vi "Main2.vi"() -> ()   [LabVIEW 2016]
panel:
  out "To send":i32
  out "Status":u16
  out "Pot 1":u16
  out "Pot 2":u16
  out "SW1 H":bool
  out "SW1 L":bool
  out "SW2 H":bool
  out "SW2 L":bool
  out "SW3 H":bool
  out "SW3 L":bool
  out "SW4 H":bool
  out "SW4 L":bool
  out "Read Status":bool[](array[boolean])
  in  "stop":bool
  out "FIFO notEmpty":bool
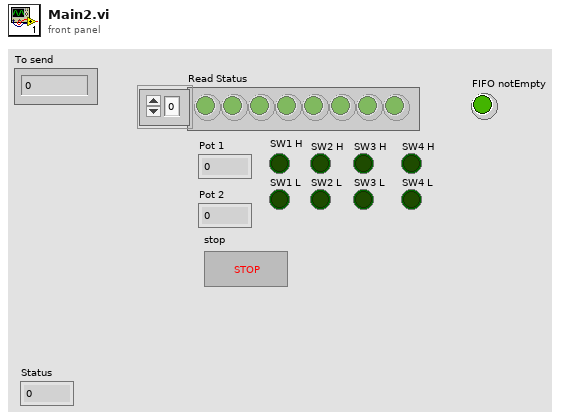
[diagram p1: front panel]
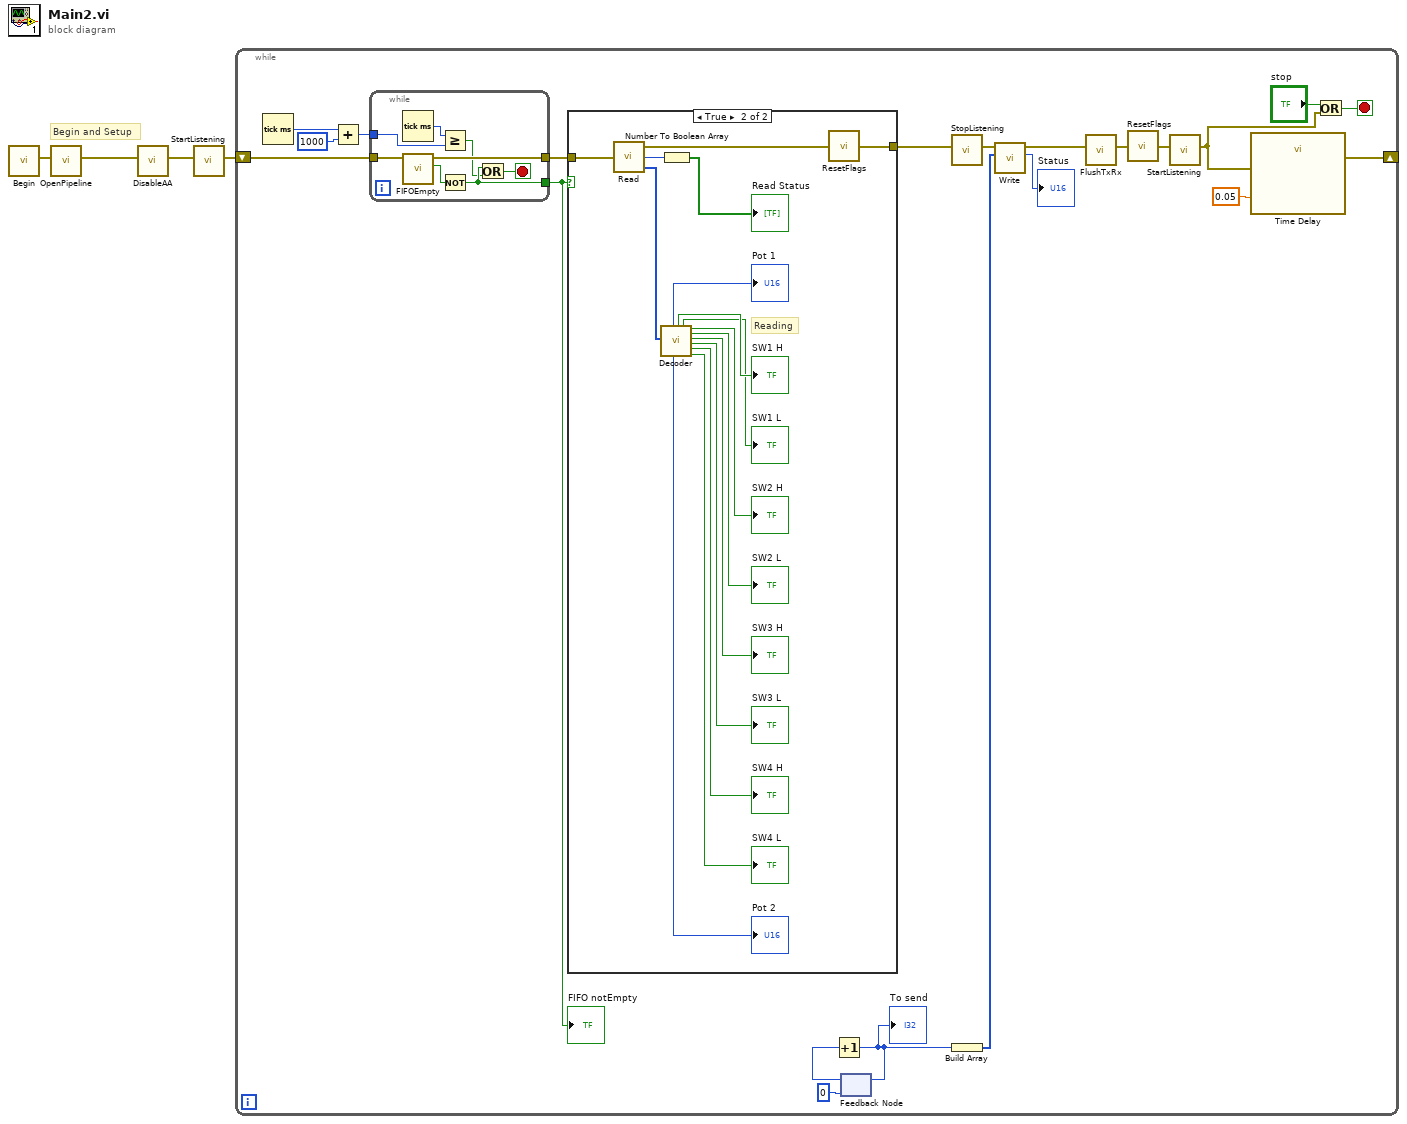
[diagram p0: block diagram]
diagram:
  # "Begin and Setup"
  n1 = call "Begin.vi"() -> ("error out"=w4:errorcluster)  [unwired: 11 in]
  n2 = call "OpenPipeline.vi"("error in (no error)"=w4) -> ("error out"=w3:errorcluster)  [unwired: 10 in]
  n3 = call "DisableAA.vi"("error in (no error)"=w3) -> ("error out"=w2:errorcluster)  [unwired: 10 in]
  n4 = call "StartListening.vi"("error in (no error)"=w2) -> ("error out"=w1:errorcluster)  [unwired: 10 in]
  n5 = while {
    shift-right: [w5] -> _
    shift-left: w1 -> [w22]
    stop <- w24 stop-if-true
    n6 = Tick Count (ms)() -> (millisecond timer value=w21:u32)
    n7 = Add(x=w21, y=u32 1000) -> (x+y=w19:u32)
    n8 = while {
      tunnel: [w33] -> w25
      tunnel: w22 -> [w32]
      tunnel: [w29] -> w8
      tunnel: w19 -> [w26]
      stop <- w30 stop-if-true
      n9 = Tick Count (ms)() -> (millisecond timer value=w28:u32)
      n10 = call "FIFOEmpty.vi"("error in (no error)"=w32) -> ("RX_EMPTY"=w31:bool, "error out"=w33:errorcluster)  [unwired: 9 in]
      n11 = Greater Or Equal?(x=w28, y=w26) -> (x >= y?=w27:bool)
      n12 = Not(x=w31) -> (.not. x?=w29:bool)
      n13 = Or(x=w29, y=w27) -> (x .or. y?=w30:bool)
    }
    "FIFO notEmpty" <- w8
    n14 = case shown="True" w8 {
      tunnel: w25 -> [w34 w36]
      tunnel: [w34 w35] -> w13
      frame False {
        # "Writing"
      }
      frame True {
        # "Reading"
        n15 = call "Read.vi"("error in (no error)"=w36) -> ("error out"=w50:errorcluster, "Status"=w38:u16, "Data frame"=w49:u16[])
        n16 = call "Decoder.vi"("Data frame"=w49) -> ("Pot 1"=→"Pot 1":u16, "Pot 2"=→"Pot 2":u16, "SW1 H"=→"SW1 H":bool, "SW1 L"=→"SW1 L":bool, "SW2 H"=→"SW2 H":bool, "SW2 L"=→"SW2 L":bool, "SW3 H"=→"SW3 H":bool, "SW3 L"=→"SW3 L":bool, "SW4 H"=→"SW4 H":bool, "SW4 L"=→"SW4 L":bool)  [unwired: 9 in]
        n17 = Number To Boolean Array(number=w38) -> (Boolean array=→"Read Status":bool[])
        n18 = call "ResetFlags.vi"("error in (no error)"=w50) -> ("error out"=w35:errorcluster)
      }
    }
    n19 = feedback #1(u32 0 ("y")) -> (w11:u32)
    n20 = Increment(x=w11) -> (x+1=w12:u32)
    "To send" <- w12
    n21 = feedback-in #1(w12) -> ()
    n22 = call "StopListening.vi"("error in (no error)"=w13) -> ("error out"=w14:errorcluster)  [unwired: 10 in]
    n23 = Build Array(w12) -> (w9:u32[])
    n24 = call "Write.vi"("array"=w9, "error in (no error)"=w14) -> ("Status"=→"Status":u16, "error out"=w15:errorcluster)  [unwired: 8 in]
    n25 = call "FlushTxRx.vi"("error in (no error)"=w15) -> ("error out"=w17:errorcluster)  [unwired: 10 in]
    n26 = call "ResetFlags.vi"("error in (no error)"=w17) -> ("error out"=w16:errorcluster)
    n27 = call "StartListening.vi"("error in (no error)"=w16) -> ("error out"=w6:errorcluster)  [unwired: 10 in]
    n28 = call "Time Delay"("error in (no error)"=w6, "Delay Time (s)"=0.05) -> ("error out"=w5:errorcluster)  [unwired: 9 in]
    n29 = Or(x="stop", y=w6) -> (x .or. y?=w24:bool)
  }
